vi "imageProfile.vi"(8 "error in (no error)":errorcluster, 10 "Point":T1, 11 "ImageStreamViewer in":refnum<class "ImageStreamViewer.lvclass">) -> (0 "error out":errorcluster, 3 "ImageStreamViewer out":refnum<class "ImageStreamViewer.lvclass">)   [LabVIEW 2011, in "Views.lvlib" / "Camera.lvlib" / "ImageStreamViewer.lvclass"]
uses:
  ImageStreamViewer.lvclass
  <vilib>/Utility/miscctls.llb/LVPoint32TypeDef.ctl
  ImageStreamViewer.lvclass/ImageStreamViewer.ctl
panel:
  # "if the user clicked inside the image,\nthen redraw the overlays and display the\nline profiles."
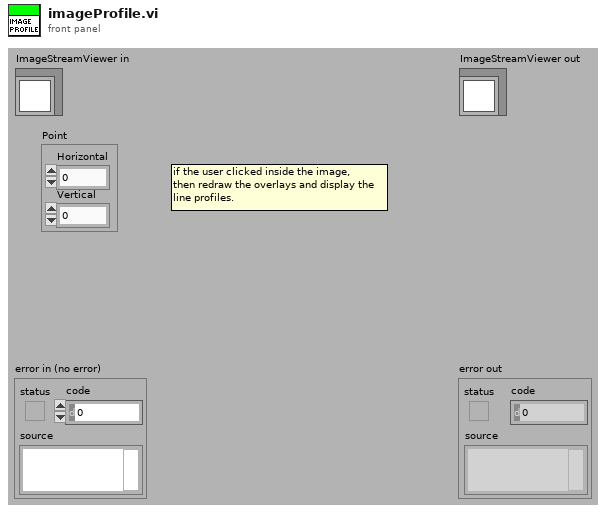
[diagram p1: front panel]
types:
  T1 = typedef "LVPoint32TypeDef.ctl" = cluster{"Horizontal":i32, "Vertical":i32}
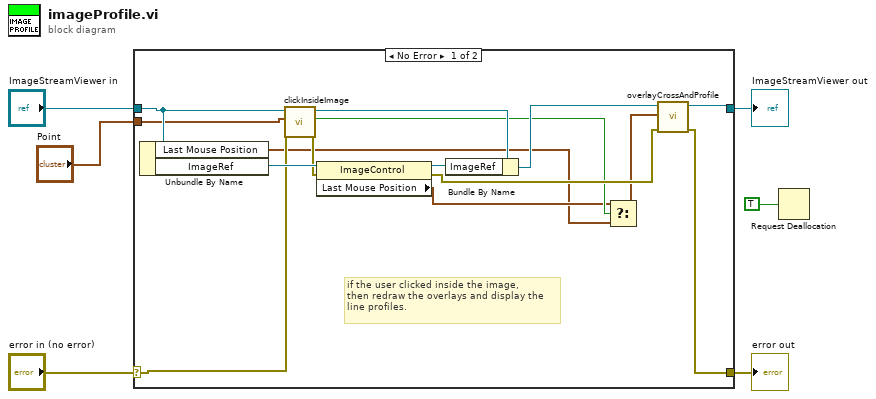
[diagram p0: block diagram]
diagram:
  n1 = case shown="No Error" "error in (no error)" {
    selector: "error in (no error)" -> [w12 w23]
    tunnel: [w17 w23] -> w5
    tunnel: [w16 w22] -> w3
    tunnel: "ImageStreamViewer in" -> [w14 w22]
    tunnel: "Point" -> [w7 _]
    frame No Error {
      # "if the user clicked inside the image,\nthen redraw the overlays and display the\nline profiles."
      n2 = Unbundle By Name(w14) -> ("Last Mouse Position"=w8:cluster{"X":i32, "Y":i32}, "ImageRef"=w21:refnum<vi>)
      n3 = call "clickInsideImage.vi"("error in (no error)"=w12, "Point"=w7, "ImageStreamViewer in"=w14) -> ("error out"=w10:errorcluster, "clickInsideImage?"=w11:bool, "ImageStreamViewer out"=w13:refnum<class "ImageStreamViewer.lvclass">)  [unwired: 6 in]
      n4 = property class="ImageControl"(reference=w21, error in=w10) -> (reference out=w20:refnum<vi>, error out=w18:errorcluster, "Last Mouse Position"=w9:cluster{"X":i32, "Y":i32})
      n5 = Bundle By Name(cluster=w13, "ImageRef"=w20) -> (w19:refnum<class "ImageStreamViewer.lvclass">)
      n6 = Select(t=w9, s=w11, f=w8) -> (s? t:f=w15:cluster{"X":i32, "Y":i32})
      n7 = call "overlayCrossAndProfile.vi"("error in (no error)"=w18, "Last Mouse P"=w15, "ImageStreamViewer in"=w19) -> ("error out"=w17:errorcluster, "ImageStreamViewer out"=w16:refnum<class "ImageStreamViewer.lvclass">)  [unwired: 7 in]
    }
    frame Error {
    }
  }
  "error out" <- w5
  "ImageStreamViewer out" <- w3
  n8 = Request Deallocation(TRUE ("flag")) -> ()
